vi "Teleop.vi"(10 "Match Info":T3={"Autonomous Elapsed Seconds"=0.0, "TeleOp Elapsed Seconds"=0.0, "Disabled Elapsed Seconds"=0.0, "Visited Autonomous"=FALSE, "Visited TeleOp"=FALSE, "Visited Disabled"=FALSE, "Autonomous Settings"={"Autonomous Style"=enum."Independent", "VI Refnum"=refnum}}, 11 "Call Context":T4) -> ()   [LabVIEW 2016]
doc: "This VI is called for each TeleOp packet received from the DS where the robot is not disabled. It is often used to read from the joysticks and update I/O or to update setpoints for timed control loops. It should complete and return within 20 milliseconds or it may miss DS packets."
uses:
  <vilib>/Rock Robotics/WPI/DriverStation/WPI_DriverStationDerivedRobotMode.ctl
  <vilib>/Rock Robotics/WPI/DriverStation/WPI_DriverStationMatch Info.ctl
  <vilib>/Rock Robotics/Network Tables/NT Read Boolean.vi
  <vilib>/Rock Robotics/Network Tables/NT Read Number.vi
  Robot Global Data.vi
  <vilib>/Rock Robotics/WPI/Utilities/WPI_GetSetVariantRefNum.vi
  <vilib>/Rock Robotics/Network Tables/NT Write Boolean Array.vi
  <vilib>/Rock Robotics/Network Tables/NT Write Numeric Array.vi
  <vilib>/Rock Robotics/Network Tables/NT Write Boolean.vi
  <vilib>/Rock Robotics/WPI/Ultrasonic/WPI_SonarMB1010AnalogRefNum Registry Get.vi
  <vilib>/Rock Robotics/WPI/Ultrasonic/WPI_SonarMB1010AnalogGetRange.vi
  2039lib.lvlib
panel:
  out "Pick Up Roller 2":dbl
  out "Agitator 2":dbl
  out "Speed of Shooter":dbl
  out "Voltage 2":dbl
  out "Voltage":dbl
  out "Toggle 7":bool
  out "Numeric 4":dbl
  out "Numeric 3":dbl
  out "Numeric 2":dbl
  out "Numeric":dbl
  out "PID gains out":T1={"proportional gain (Kc)"=1.0, "integral time (Ti, min)"=0.01, "derivative time (Td, min)"=0.0} {"derivative time (Td, min)" format="%.3f"; "integral time (Ti, min)" format="%.3f"; "proportional gain (Kc)" format="%.3f"}
  in  "PID gains":T1={"proportional gain (Kc)"=1.0, "integral time (Ti, min)"=0.01, "derivative time (Td, min)"=0.0} {"derivative time (Td, min)" format="%.3f"; "integral time (Ti, min)" format="%.3f"; "proportional gain (Kc)" format="%.3f"}
  in  "Teleop State":T2(ring)
  out "Toggle 6":bool
  out "Toggle 5":bool
  out "Toggle 4":bool
  out "Toggle 3":bool
  out "Toggle 2":bool
  out "Sample Slider 0":dbl(slide) scale=0.0..5.0
  out "Sample Boolean 1":bool
  out "Sample Boolean 0":bool
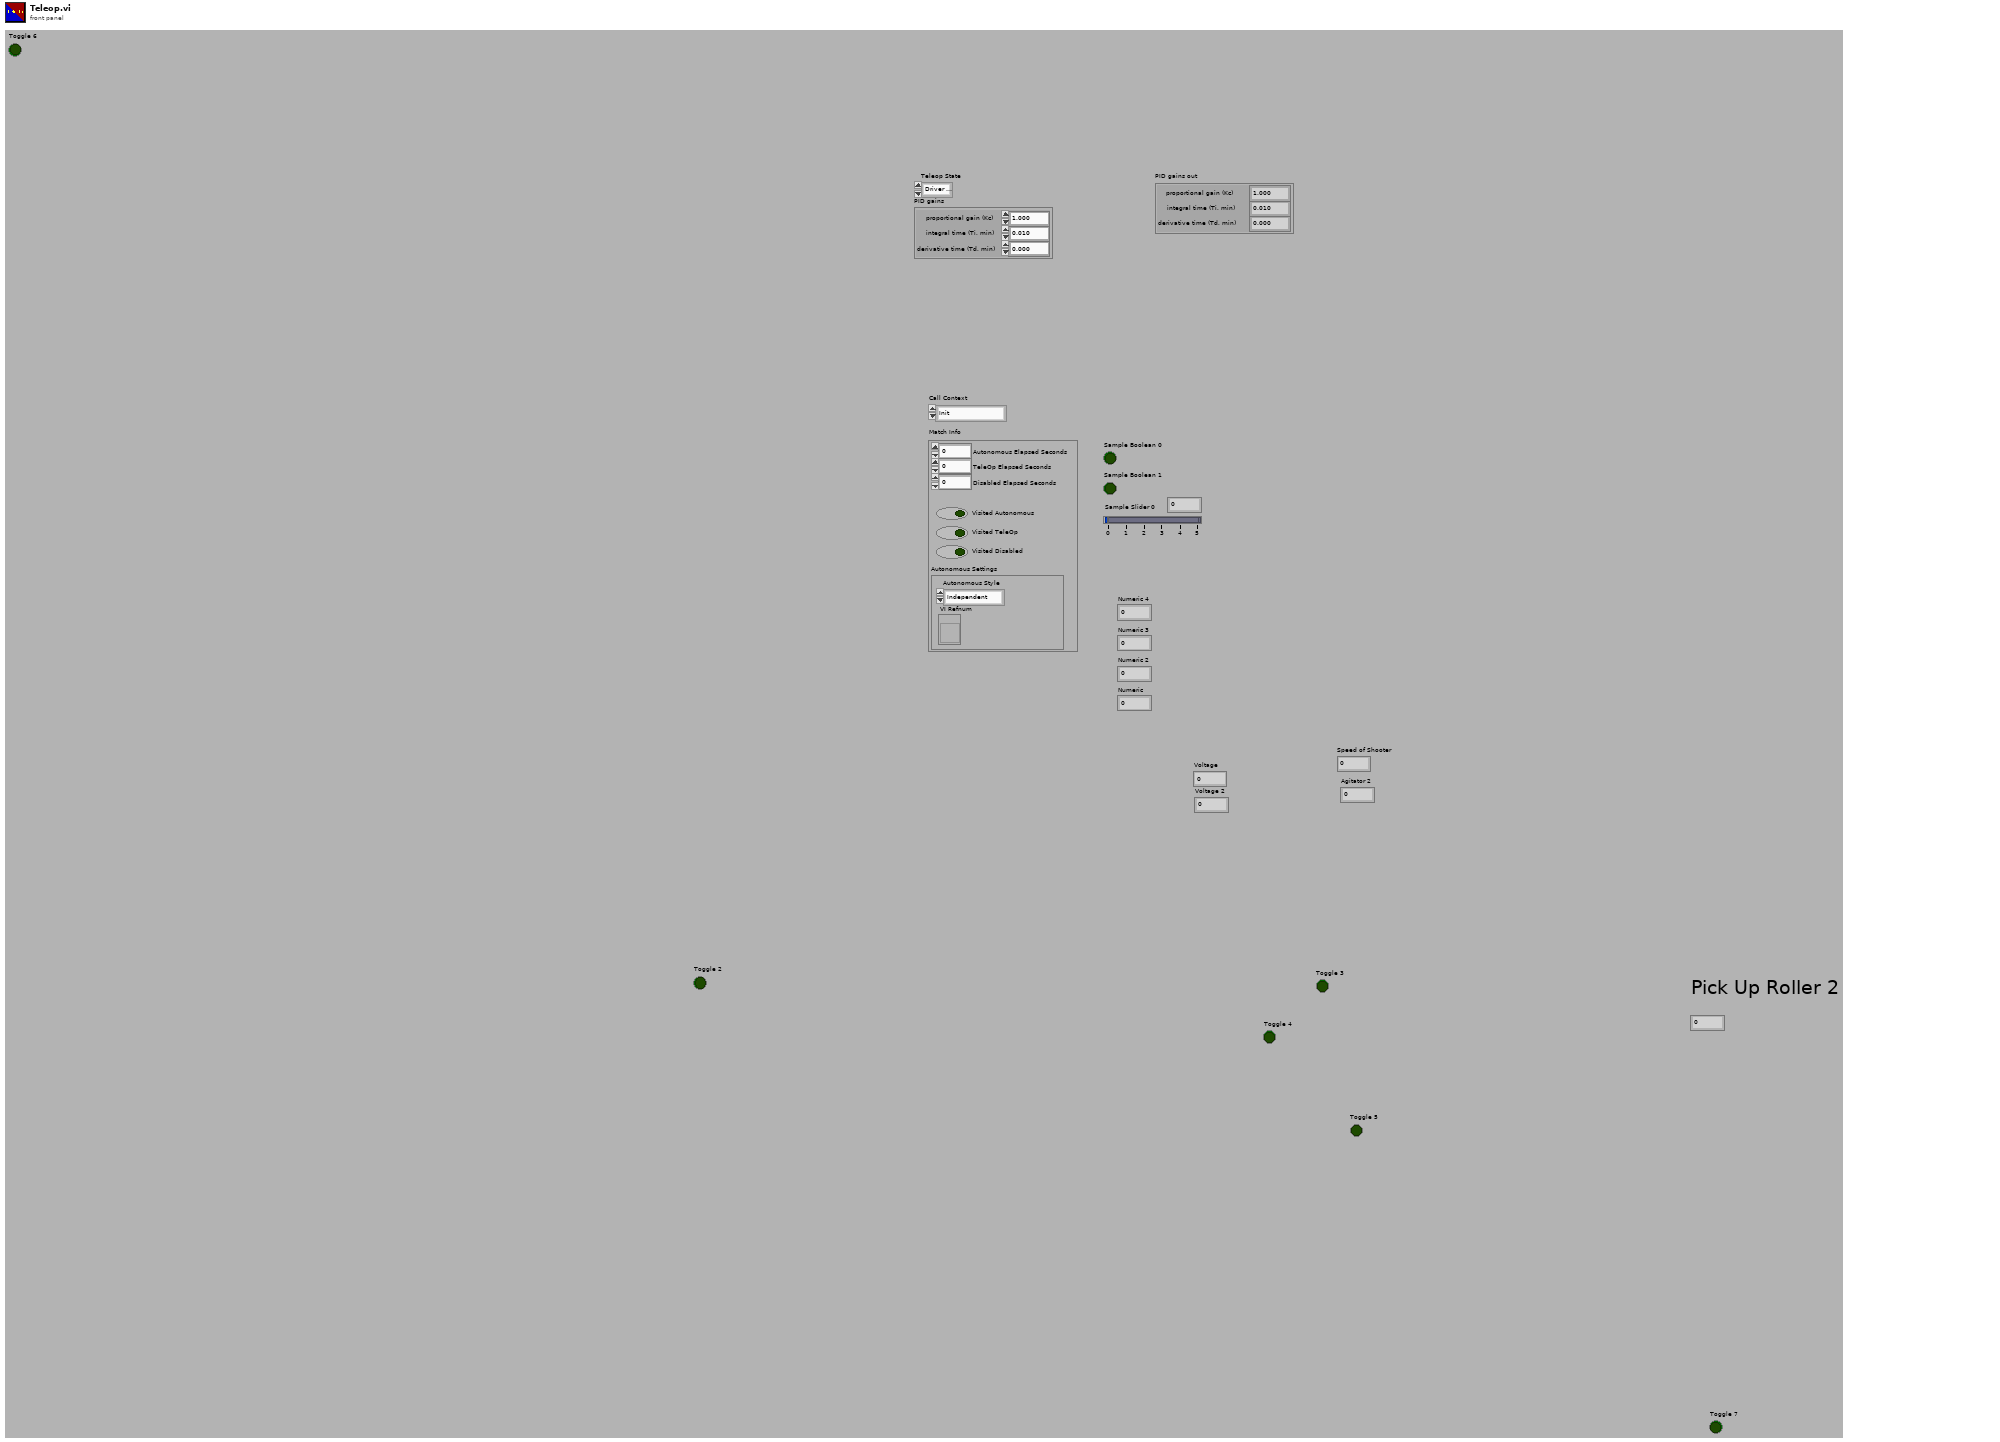
[diagram p1: front panel]
types:
  T1 = cluster{"proportional gain (Kc)":dbl, "integral time (Ti, min)":dbl, "derivative time (Td, min)":dbl}
  T2 = enum16{"Driver Control", "PID Autotune", "Gear Coarse Adjust", "Gear Fine Adjust"}
  T3 = typedef "WPI_DriverStationMatch Info.ctl" = cluster{"Autonomous Elapsed Seconds":dbl, "TeleOp Elapsed Seconds":dbl, "Disabled Elapsed Seconds":dbl, "Visited Autonomous":bool, "Visited TeleOp":bool, "Visited Disabled":bool, "Autonomous Settings":cluster{"Autonomous Style":enum16{"Iterative", "Independent"}, "VI Refnum":refnum<vi>}}
  T4 = typedef "WPI_DriverStationDerivedRobotMode.ctl" = enum16{"Init", "Execute", "Stop"}
  T5 = typedef "WPI_MotorControlDeviceRef.ctl" = cluster{"DeviceStatus":errorcluster, "Type":T6, "PWM":cluster{"PWM Channel":T7, "DeadBand":T8}, "CAN":cluster{"Device Number":u8, "SetOutput VI Ref":variant, "GetOutput VI Ref":variant, "Enable VI Ref":variant, "Disable VI Ref":variant, "Data":variant}, "Invert":bool}
  T6 = typedef "WPI_MotorControlType.ctl" = enum16{"PWM", "CAN"}
  T7 = typedef "FPGA_DIOPWMChannel.ctl" = enum8{"PWM 0", "PWM 1", "PWM 2", "PWM 3", "PWM 4", "PWM 5", "PWM 6", "PWM 7", "PWM 8", "PWM 9", "PWM MXP 0", "PWM MXP 1", "PWM MXP 2", "PWM MXP 3", "PWM MXP 4", "PWM MXP 5", "PWM MXP 6", "PWM MXP 7", "PWM MXP 8", "PWM MXP 9", "Invalid"}
  T8 = typedef "WPI_PWMDeadband.ctl" = cluster{"Name":string, "maxPositivePwm":i32, "minPositivePwm":i32, "centerPwm":i32, "maxNegativePwm":i32, "minNegativePwm":i32, "angularRange":u16}
  T9 = enum16{"Driver Control", "Gear Coarse Adjust", "Gear Fine Adjust"}
  T10 = typedef "WPI_JoystickDevRef.ctl" = cluster{"Device":T11}
  T11 = typedef "WPI_JoystickDeviceEnum.ctl" = enum16{"USB 0", "USB 1", "USB 2", "USB 3", "USB 4", "USB 5"}
  T12 = cluster{"Buttons[0]":bool, "Buttons[1]":bool, "Buttons[2]":bool, "Buttons[3]":bool, "Buttons[4]":bool, "Buttons[5]":bool, "Buttons[6]":bool, "Buttons[7]":bool, "Buttons[8]":bool, "Buttons[9]":bool, "Buttons[10]":bool, "Buttons[11]":bool, "Buttons[12]":bool}
  T13 = typedef "WPI_RobotDriveDevRef.ctl" = cluster{"DevStatus":errorcluster, "Motors[]":T5[], "Square Inputs":bool, "Max Output":dbl}
  T14 = cluster{"Buttons[0]":bool, "Buttons[1]":bool, "Buttons[2]":bool, "Buttons[3]":bool, "Buttons[4]":bool, "Buttons[5]":bool, "Buttons[6]":bool, "Buttons[7]":bool, "Buttons[8]":bool}
  T15 = typedef "WPI_ServoDeviceRef.ctl" = cluster{"DeviceStatus":errorcluster, "PWM Channel":T7, "DeadBand":T8}
  T16 = typedef "WPI_SonarMB1010AnalogDeviceRef.ctl" = cluster{"AIDeviceRef":T17, "Scaling factor (V/in)":dbl, "Average Bits":u8}
  T17 = typedef "WPI_AnalogChannelDevRef.ctl" = cluster{"DevStatus":errorcluster, "Analog Channel":T18}
  T18 = typedef "FPGA_AIChannel.ctl" = enum8{"AI 0", "AI 1", "AI 2", "AI 3", "AI MXP 0", "AI MXP 1", "AI MXP 2", "AI MXP 3", "Invalid"}
  T19 = typedef "WPI_DigitalInputDevRef.ctl" = cluster{"DevStatus":errorcluster, "DIO Channel":T20}
  T20 = typedef "FPGA_DIOChannel.ctl" = enum8{"DIO 0", "DIO 1", "DIO 2", "DIO 3", "DIO 4", "DIO 5", "DIO 6", "DIO 7", "DIO 8", "DIO 9", "DIO MXP 0", "DIO MXP 1", "DIO MXP 2", "DIO MXP 3", "DIO MXP 4", "DIO MXP 5", "DIO MXP 6", "DIO MXP 7", "DIO MXP 8", "DIO MXP 9", "DIO MXP 10", "DIO MXP 11", "DIO MXP 12", "DIO MXP 13", "DIO MXP 14", "DIO MXP 15", "SPI Port CS1", "SPI Port CS2", "SPI Port CS3", "SPI Port MISO", "SPI Port MOSI", "Invalid"}
  T21 = typedef "WPI_SwitchDevRef.ctl" = cluster{"DevStatus":errorcluster, "DIO Channel":T20, "CntIndex":T22, "Normally Closed":bool}
  T22 = typedef "FPGA_CounterCtrSystemIndex.ctl" = enum8{"Ctr 0", "Ctr 1", "Ctr 2", "Ctr 3", "Ctr 4", "Ctr 5", "Ctr 6", "Ctr 7", "Invalid"}
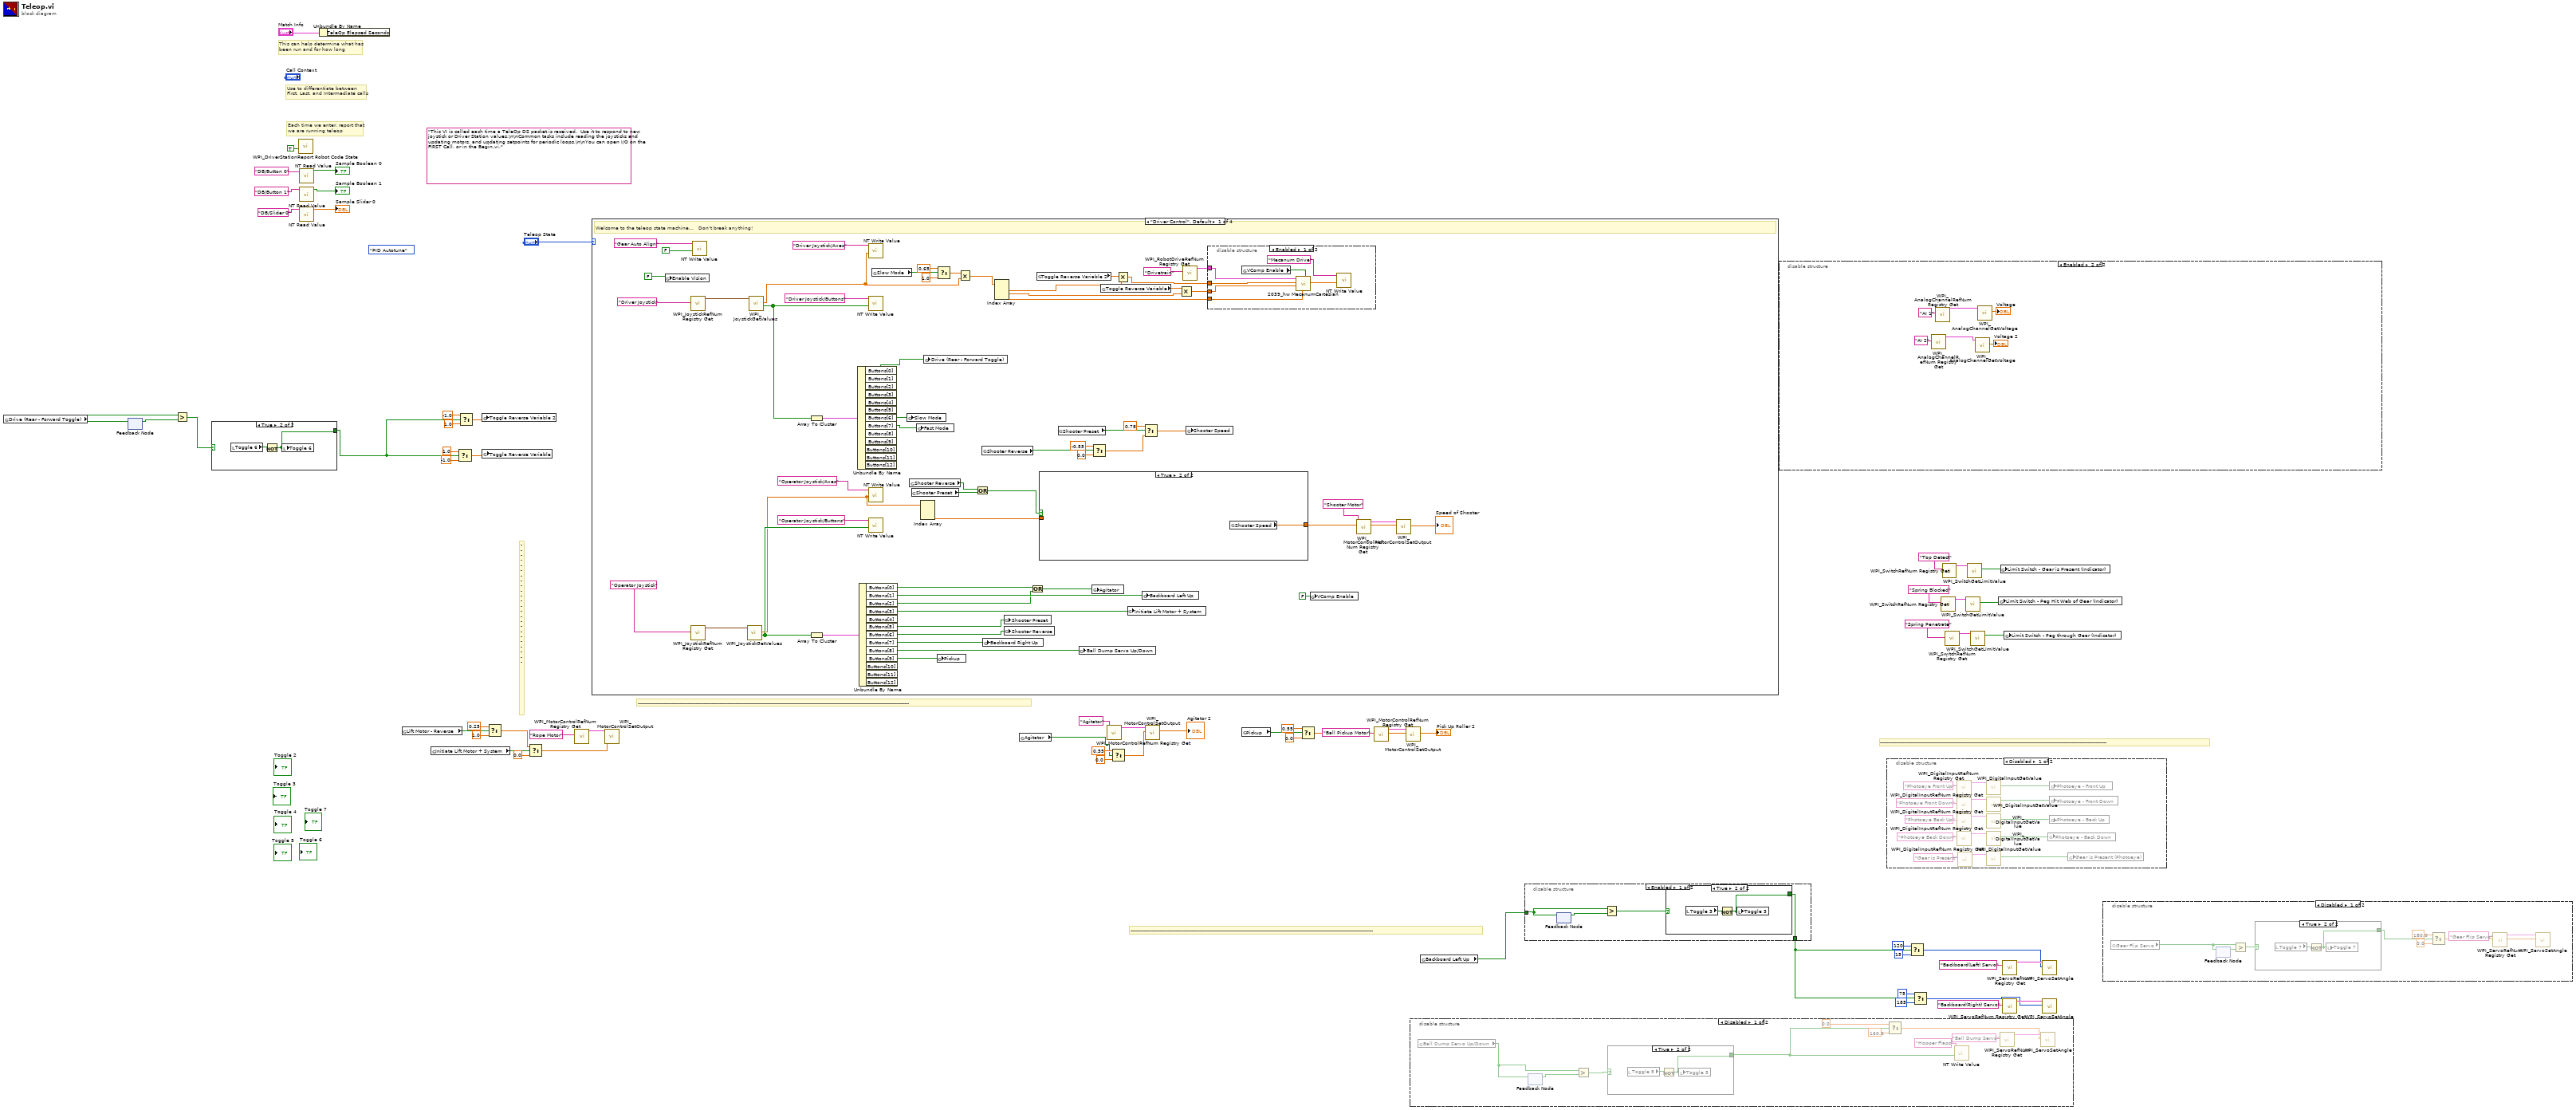
[diagram p0: block diagram]
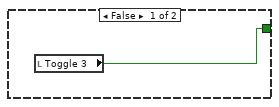
[diagram p3: hidden frame]
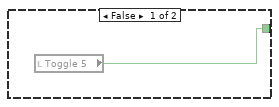
[diagram p5: hidden frame]
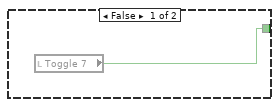
[diagram p7: hidden frame]
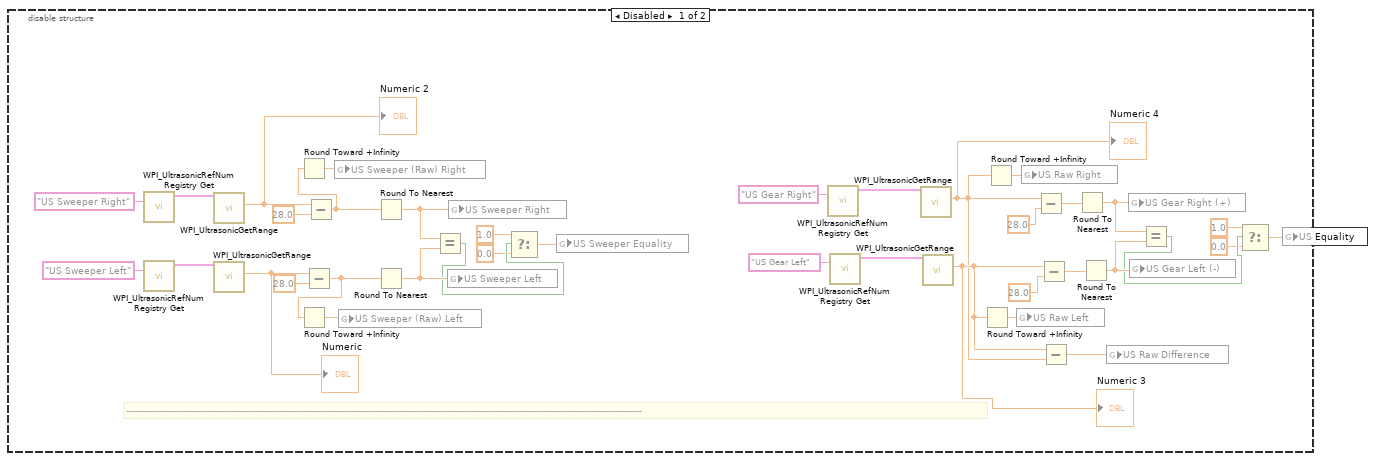
[diagram p9: hidden frame]
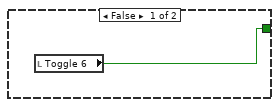
[diagram p10: hidden frame]
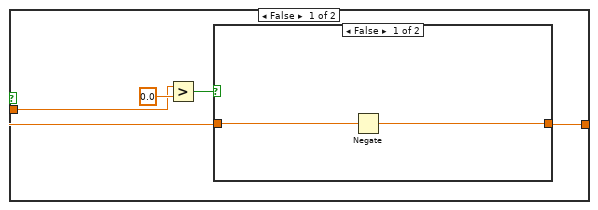
[diagram p11: hidden frame]
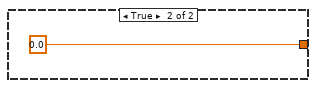
[diagram p12: hidden frame]
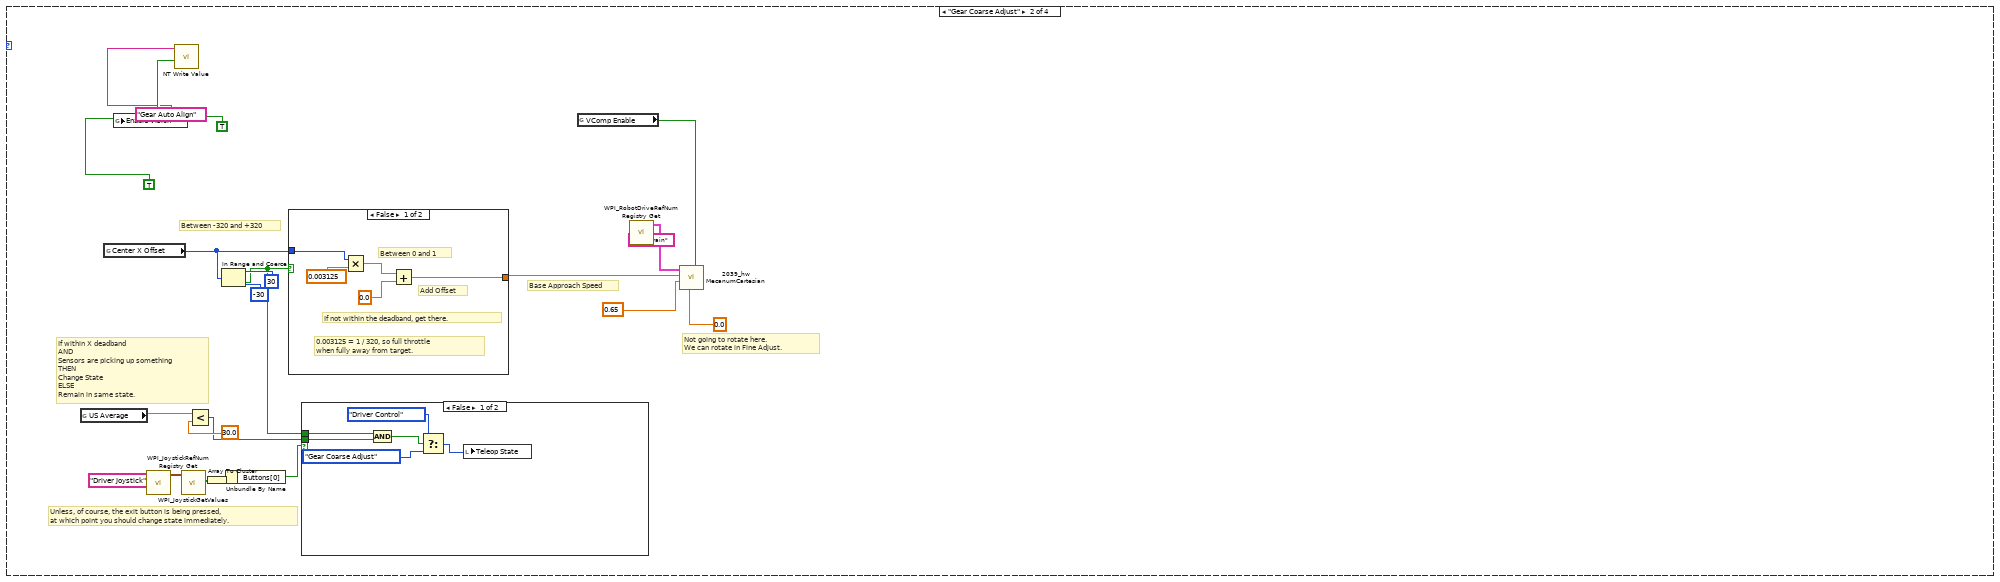
[diagram p14: hidden frame]
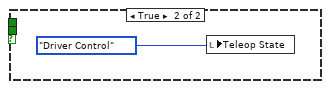
[diagram p15: hidden frame]
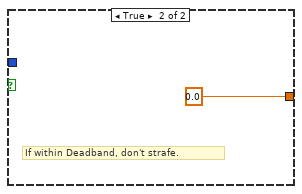
[diagram p16: hidden frame]
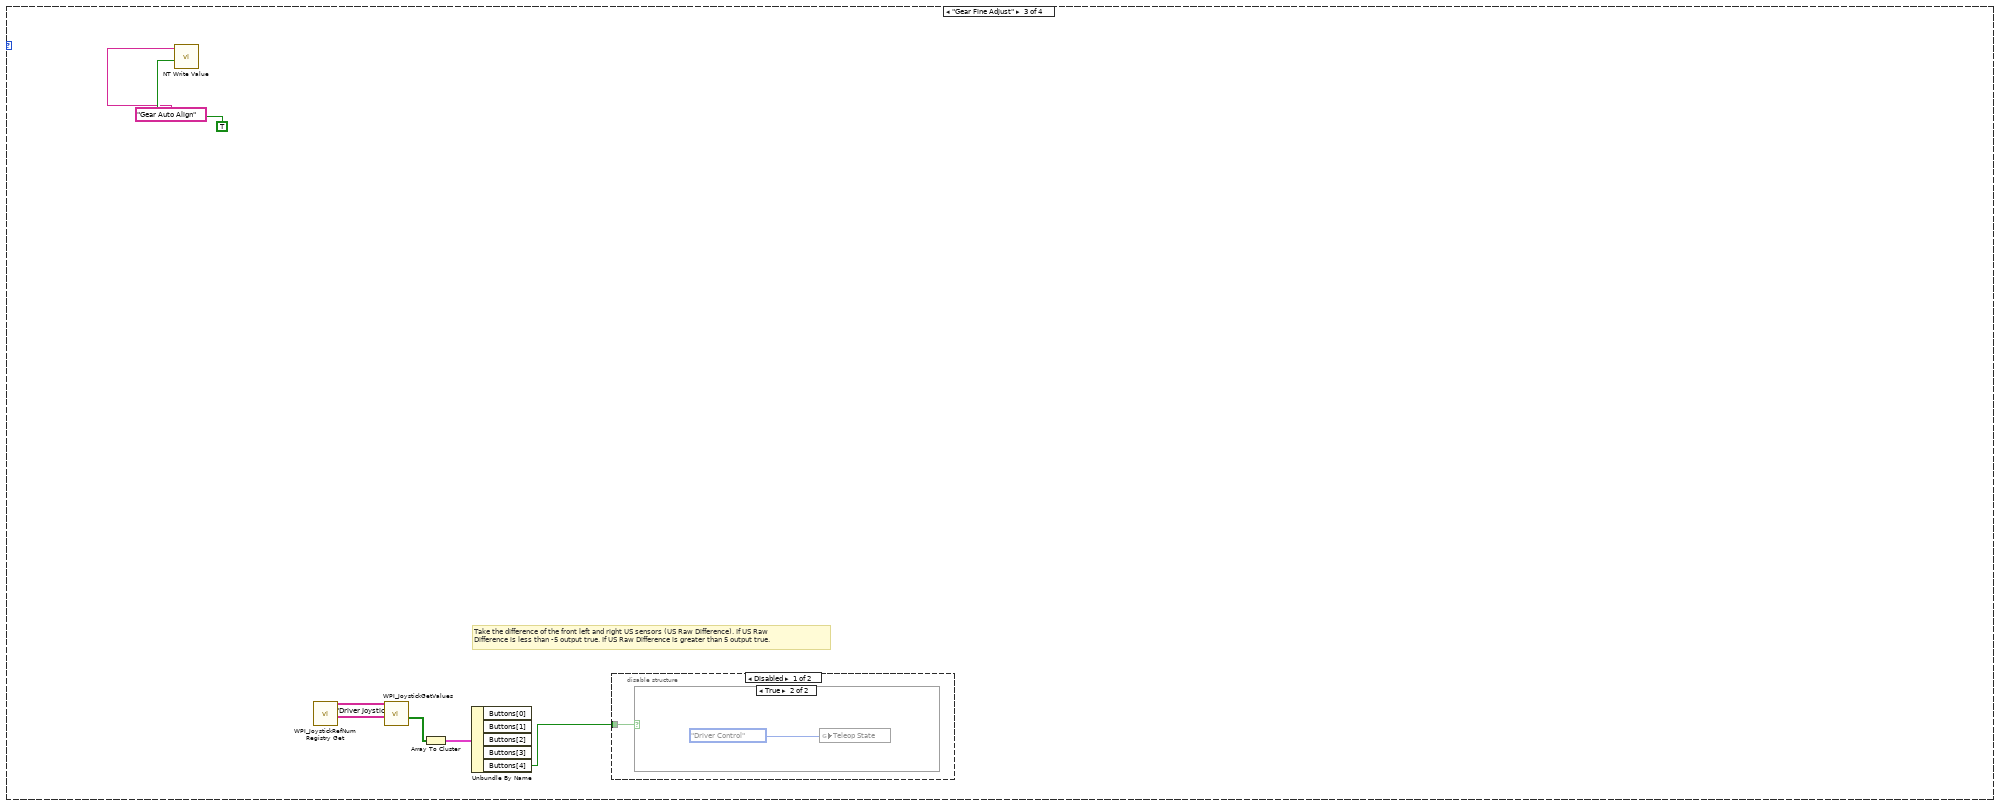
[diagram p17: hidden frame]
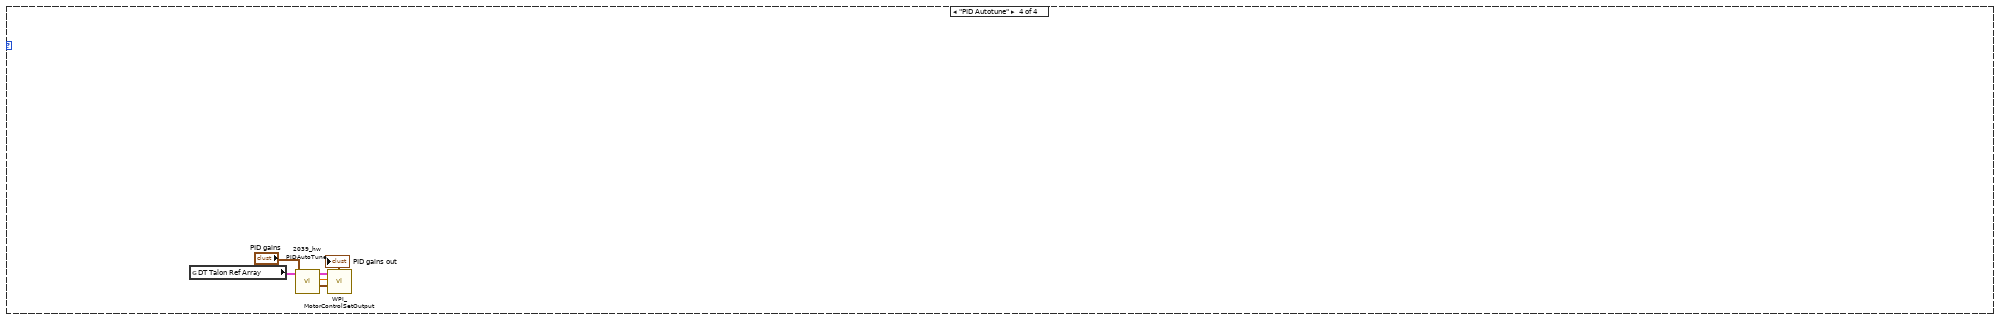
[diagram p20: hidden frame]
diagram:
  (unwired) T2."PID Autotune" ("Teleop State")
  (unwired) "This VI is called each time a TeleOp DS packet is received.  Use it to respond to new joystick or Driver Station values.\n\nCommon tasks include reading the joysticks and updating motors, and updating setpoints for periodic loops.\n\nYou can open I/O on the FIRST Call, or in the Begin.vi."
  # "-\n-\n-\n-\n-\n-\n-\n-\n-\n-\n-\n-\n-\n-\n-\n-\n-\n-\n-\n-\n-\n-\n-\n-"
  # "--------------------------------------------------------------------------------------------------------------------------------------------------------------------------"
  # "--------------------------------------------------------------------------------------------------------------------------------------------------------"
  # "----------------------------------------------------------------------------------------------------------------------------------------------"
  # "Each time we enter, report that\nwe are running teleop"
  # "Use to differentiate between\nFirst, Last, and Intermediate calls"
  # "This can help determine what has\nbeen run and for how long"
  n1 = global read "Robot Global Data.vi" "Drive (Rear - Forward Toggle)"() -> (w3:bool)
  n2 = feedback #1() -> (w35:bool)  [unwired: 1 in]
  n3 = feedback-in #1(w3) -> ()
  n4 = Greater?(x=w3, y=w35) -> (0:w34:bool)
  n5 = case shown="True" w34 {
    tunnel: [w64 w65] -> w7
    frame False {
      n6 = local read "Toggle 6"() -> (w64:bool)
    }
    frame True {
      n7 = local read "Toggle 6"() -> (w66:bool)
      n8 = Not(x=w66) -> (.not. x?=w65:bool)
      n9 = local write "Toggle 6"(w65) -> ()
    }
  }
  n10 = call <vilib>:"WPI_DriverStationReport Robot Code State.vi"("TeleOp"=TRUE ("Autonomous")) -> ()  [unwired: 10 in, 1 out]
  n11 = call-poly <vilib>:"NT Read Value.vi"("Name"="DB/Button 0" ("refnum name")) -> ("Boolean"=→"Sample Boolean 0":bool)  [unwired: 9 in, 1 out]
  n12 = call-poly <vilib>:"NT Read Value.vi"("Name"="DB/Button 1" ("refnum name")) -> ("Boolean"=→"Sample Boolean 1":bool)  [unwired: 9 in, 1 out]
  n13 = call-poly <vilib>:"NT Read Value.vi"("Name"="DB/Slider 0" ("refnum name")) -> ("Numeric"=→"Sample Slider 0":dbl)  [unwired: 9 in, 1 out]
  n14 = Unbundle By Name("Match Info") -> ()  [unwired: 1 out]
  n15 = global read "Robot Global Data.vi" "Lift Motor - Reverse"() -> (w26:bool)
  n16 = global read "Robot Global Data.vi" "Initiate Lift Motor + System"() -> (w31:bool)
  n17 = Select(t=1.0, s=w7, f=-1.0) -> (s? t:f=w44:dbl)
  n18 = Select(t=-1.0, s=w7, f=1.0) -> (s? t:f=w10:dbl)
  n19 = global write "Robot Global Data.vi" "Toggle Reverse Variable 2"(w10) -> ()
  n20 = global write "Robot Global Data.vi" "Toggle Reverse Variable"(w44) -> ()
  n21 = Select(t=0.25, s=w26, f=1.0) -> (s? t:f=w29:dbl)
  n22 = Select(t=w29, s=w31, f=0.0) -> (s? t:f=w36:dbl)
  n23 = call <vilib>:"WPI_MotorControlRefNum Registry Get.vi"("refnum name"="Rope Motor") -> ("MotorControlDevRef"=w48:T5)  [unwired: 9 in, 1 out]
  n24 = case shown="\"Driver Control\", Default" "Teleop State" {
    frame "Driver Control", Default {
      # "Welcome to the teleop state machine...   Don't break anything!"
      n25 = global write "Robot Global Data.vi" "Enable Vision"(FALSE) -> ()
      n26 = call <vilib>:"WPI_JoystickRefNum Registry Get.vi"("refnum name"="Driver Joystick") -> ("JoystickDevRef"=w123:T10)  [unwired: 1 in, 9 out]
      n27 = call <vilib>:"WPI_JoystickRefNum Registry Get.vi"("refnum name"="Operator Joystick") -> ("JoystickDevRef"=w118:T10)  [unwired: 9 in, 1 out]
      n28 = call-poly <vilib>:"NT Write Value.vi"("Boolean"=FALSE, "Name"="Gear Auto Align") -> ()  [unwired: 9 in, 1 out]
      n29 = call <vilib>:"WPI_JoystickGetValues.vi"("JoystickDevRef"=w118) -> ("Buttons"=w115:bool[], "Axes"=w94:dbl[])  [unwired: 6 in, 3 out]
      n30 = call <vilib>:"WPI_JoystickGetValues.vi"("JoystickDevRef"=w123) -> ("Buttons"=w120:bool[], "Axes"=w97:dbl[])  [unwired: 6 in, 3 out]
      n31 = Array To Cluster(array=w120) -> (cluster=w111:T12)
      n32 = Array To Cluster(array=w115) -> (cluster=w112:T12)
      n33 = Unbundle By Name(w111) -> ("Buttons[0]"=w110:bool, "Buttons[6]"=w107:bool, "Buttons[7]"=w104:bool)  [unwired: 10 out]
      n34 = Unbundle By Name(w112) -> ("Buttons[0]"=w71:bool, "Buttons[1]"=w90:bool, "Buttons[2]"=w72:bool, "Buttons[3]"=w87:bool, "Buttons[5]"=w85:bool, "Buttons[6]"=w84:bool, "Buttons[7]"=w109:bool, "Buttons[8]"=w108:bool, "Buttons[9]"=w67:bool)  [unwired: 4 out]
      n35 = call-poly <vilib>:"NT Write Value.vi"("Numeric Array"=w97, "Name"="Driver Joystick/Axes") -> ()  [unwired: 9 in, 1 out]
      n36 = call-poly <vilib>:"NT Write Value.vi"("Boolean Array"=w120, "Name"="Driver Joystick/Buttons") -> ()  [unwired: 9 in, 1 out]
      n37 = call-poly <vilib>:"NT Write Value.vi"("Numeric Array"=w94, "Name"="Operator Joystick/Axes") -> ()  [unwired: 9 in, 1 out]
      n38 = call-poly <vilib>:"NT Write Value.vi"("Boolean Array"=w115, "Name"="Operator Joystick/Buttons") -> ()  [unwired: 9 in, 1 out]
      n39 = global read "Robot Global Data.vi" "Slow Mode"() -> (w101:bool)
      n40 = global write "Robot Global Data.vi" "Slow Mode"(w107) -> ()
      n41 = global read "Robot Global Data.vi" "Shooter Reverse"() -> (w75:bool)
      n42 = global read "Robot Global Data.vi" "Shooter Preset"() -> (w76:bool)
      n43 = global write "Robot Global Data.vi" "Fast Mode"(w104) -> ()
      n44 = Index Array(array=w94) -> (element #3=w88:dbl)  [unwired: 3 in, 2 out]
      n45 = global write "Robot Global Data.vi" "Drive (Rear - Forward Toggle)"(w110) -> ()
      n46 = Select(t=0.65, s=w101, f=1.0) -> (s? t:f=w98:dbl)
      n47 = global write "Robot Global Data.vi" "Pickup"(w67) -> ()
      n48 = Multiply(x=w98, y=w97) -> (x*y=w96:dbl[])
      n49 = Or(x=w75, y=w76) -> (x .or. y?=w74:bool)
      n50 = global read "Robot Global Data.vi" "Shooter Reverse"() -> (w80:bool)
      n51 = global write "Robot Global Data.vi" "Backboard Right Up"(w109) -> ()
      n52 = Index Array(array=w96) -> (element #1=w69:dbl, element #2=w103:dbl, element #3=w102:dbl)  [unwired: 3 in]
      n53 = global write "Robot Global Data.vi" "Shooter Preset"(w85) -> ()
      n54 = global write "Robot Global Data.vi" "Shooter Reverse"(w84) -> ()
      n55 = Or(x=w71, y=w72) -> (x .or. y?=w73:bool)
      n56 = global read "Robot Global Data.vi" "Toggle Reverse Variable 2"() -> (w70:dbl)
      n57 = case shown="True" w74 {
        tunnel: [w128 w134] -> w89
        tunnel: w88 -> [w127 _]
        frame False {
          n58 = Greater?(x=w127, y=0.0) -> (0:w129:bool)
          n59 = case shown="False" w129 {
            tunnel: [w131 0.0 ("y")] -> w128
            tunnel: w127 -> [w132 _]
            frame False {
              n60 = Negate(x=w132) -> (-x=w131:dbl)
            }
            frame True {
            }
          }
        }
        frame True {
          n61 = global read "Robot Global Data.vi" "Shooter Speed"() -> (w134:dbl)
        }
      }
      n62 = global read "Robot Global Data.vi" "Shooter Preset"() -> (w83:bool)
      n63 = global write "Robot Global Data.vi" "Ball Dump Servo Up/Down"(w108) -> ()
      n64 = Select(t=-0.55, s=w80, f=0.0) -> (s? t:f=w77:dbl)
      n65 = global write "Robot Global Data.vi" "Agitator"(w73) -> ()
      n66 = global read "Robot Global Data.vi" "Toggle Reverse Variable"() -> (w113:dbl)
      n67 = Multiply(x=w70, y=w69) -> (x*y=w68:dbl)
      n68 = global write "Robot Global Data.vi" "Initiate Lift Motor + System"(w87) -> ()
      n69 = global write "Robot Global Data.vi" "Backboard Left Up"(w90) -> ()
      n70 = Select(t=0.78, s=w83, f=w77) -> (s? t:f=w81:dbl)
      n71 = Multiply(x=w113, y=w103) -> (x*y=w114:dbl)
      n72 = call <vilib>:"WPI_RobotDriveRefNum Registry Get.vi"("refnum name"="Drivetrain") -> ("RobotDriveDevRef"=w125:T13)  [unwired: 1 in, 9 out]
      n73 = global write "Robot Global Data.vi" "Shooter Speed"(w81) -> ()
      n74 = disable-structure shown="Enabled" {
        disable-tunnel: w125 -> [w141 _]
        disable-tunnel: w114 -> [w138 _]
        disable-tunnel: w102 -> [w135 _]
        disable-tunnel: w68 -> [w136 _]
        frame Enabled {
          n75 = global read "Robot Global Data.vi" "VComp Enable"() -> (w137:bool)
          n76 = call "2039_hw MecanumCartesian.vi"("VComp Scaling"=w137, "Rotation"=w135, "Y"=w138, "X"=w136, "RobotDriveDevRef"=w141) -> ("Motor Values"=w139:dbl[])  [unwired: 4 in, 2 out]
          n77 = call-poly <vilib>:"NT Write Value.vi"("Numeric Array"=w139, "Name"="Mecanum Drive") -> ()  [unwired: 9 in, 1 out]
        }
        frame Disabled {
        }
      }
      n78 = global write "Robot Global Data.vi" "VComp Enable"(FALSE ("VComp Enable")) -> ()
      n79 = call <vilib>:"WPI_MotorControlRefNum Registry Get.vi"("refnum name"="Shooter Motor") -> ("MotorControlDevRef"=w92:T5)  [unwired: 9 in, 1 out]
      n80 = call <vilib>:"WPI_MotorControlSetOutput.vi"("Output"=w89, "MotorControlDevRef"=w92) -> ("Motor Output"=→"Speed of Shooter":dbl)  [unwired: 7 in, 2 out]
    }
    frame "Gear Coarse Adjust" {
      # "Base Approach Speed"
      # "If within X deadband\nAND\nSensors are picking up something\nTHEN\nChange State\nELSE\nRemain in same state."
      # "Unless, of course, the exit button is being pressed, \nat which point you should change state immediately."
      # "Not going to rotate here.\nWe can rotate in Fine Adjust."
      # "Between -320 and +320"
      n81 = global read "Robot Global Data.vi" "US Average"() -> (w150:dbl)
      n82 = global read "Robot Global Data.vi" "Center X Offset"() -> (w159:i32)
      n83 = global write "Robot Global Data.vi" "Enable Vision"(TRUE) -> ()
      n84 = call <vilib>:"WPI_JoystickRefNum Registry Get.vi"("refnum name"="Driver Joystick") -> ("JoystickDevRef"=w146:T10)  [unwired: 1 in, 9 out]
      n85 = call-poly <vilib>:"NT Write Value.vi"("Boolean"=TRUE, "Name"="Gear Auto Align") -> ()  [unwired: 9 in, 1 out]
      n86 = call <vilib>:"WPI_JoystickGetValues.vi"("JoystickDevRef"=w146) -> ("Buttons"=w145:bool[])  [unwired: 6 in, 4 out]
      n87 = Less?(x=w150, y=30.0) -> (x < y?=w148:bool)
      n88 = Array To Cluster(array=w145) -> (cluster=w144:T14)
      n89 = In Range and Coerce(upper limit=30, x=w159, lower limit=-30) -> (In Range?=w151:bool)  [unwired: 1 out]
      n90 = Unbundle By Name(w144) -> ("Buttons[0]"=w143:bool)
      n91 = case shown="False" w151 {
        tunnel: w159 -> [w174 _]
        tunnel: [w170 0.0] -> w156
        frame False {
          # "0.003125 = 1 / 320, so full throttle\nwhen fully away from target."
          # "If not within the deadband, get there."
          # "Add Offset"
          # "Between 0 and 1"
          n92 = Multiply(x=w174, y=0.003125) -> (x*y=w172:dbl)
          n93 = Add(x=w172, y=0.0) -> (x+y=w170:dbl)
        }
        frame True {
          # "If within Deadband, don't strafe."
        }
      }
      n94 = case shown="False" w143 {
        tunnel: w151 -> [w168 _]
        tunnel: w148 -> [w167 _]
        frame False {
          n95 = And(x=w168, y=w167) -> (x .and. y?=w164:bool)
          n96 = Select(t=T2."Driver Control" ("Teleop State"), s=w164, f=T2."Gear Coarse Adjust" ("Teleop State")) -> (s? t:f=w163:T2)
          n97 = local write "Teleop State"(w163) -> ()
        }
        frame True {
          n98 = local write "Teleop State"(T2."Driver Control" ("Teleop State")) -> ()
        }
      }
      n99 = global read "Robot Global Data.vi" "VComp Enable"() -> (w152:bool)
      n100 = call <vilib>:"WPI_RobotDriveRefNum Registry Get.vi"("refnum name"="Drivetrain") -> ("RobotDriveDevRef"=w154:T13)  [unwired: 1 in, 9 out]
      n101 = call "2039_hw MecanumCartesian.vi"("VComp Scaling"=w152, "Rotation"=0.0, "Y"=0.65, "X"=w156, "RobotDriveDevRef"=w154) -> ()  [unwired: 4 in, 3 out]
    }
    frame "Gear Fine Adjust" {
      # "Take the difference of the front left and right US sensors (US Raw Difference). If US Raw \nDifference is less than -5 output true. If US Raw Difference is greater than 5 output true."
      n102 = call-poly <vilib>:"NT Write Value.vi"("Boolean"=TRUE, "Name"="Gear Auto Align") -> ()  [unwired: 9 in, 1 out]
      n103 = call <vilib>:"WPI_JoystickRefNum Registry Get.vi"("refnum name"="Driver Joystick") -> ("JoystickDevRef"=w180:T10)  [unwired: 9 in, 1 out]
      n104 = call <vilib>:"WPI_JoystickGetValues.vi"("JoystickDevRef"=w180) -> ("Buttons"=w179:bool[])  [unwired: 6 in, 4 out]
      n105 = Array To Cluster(array=w179) -> (cluster=w178:T14)
      n106 = Unbundle By Name(w178) -> ("Buttons[4]"=w177:bool)  [unwired: 4 out]
      n107 = disable-structure shown="Disabled" {
        disable-tunnel: w177 -> [w183 _]
        frame Disabled {
          n108 = case shown="True" w183 {
            frame False {
            }
            frame True {
              n109 = global write "Robot Global Data.vi" "Teleop State"(T9."Driver Control") -> ()
            }
          }
        }
        frame Enabled {
        }
      }
    }
    frame "PID Autotune" {
      n110 = global read "Robot Global Data.vi" "DT Talon Ref Array"() -> (w189:T5[])
      n111 = call "2039_hw PIDAutoTune.vi"("PID gains"="PID gains", "CAN Talon SRX Ref"=w189) -> ("PID gains out"=→"PID gains out":T1, "To Motors"=w187:dbl, "Tuning Talon"=w188:T5)  [unwired: 7 in]
      n112 = call <vilib>:"WPI_MotorControlSetOutput.vi"("Output"=w187, "MotorControlDevRef"=w188) -> ()  [unwired: 7 in, 3 out]
    }
  }
  n113 = call <vilib>:"WPI_MotorControlSetOutput.vi"("Output"=w36, "MotorControlDevRef"=w48) -> ()  [unwired: 7 in, 3 out]
  n114 = global read "Robot Global Data.vi" "Agitator"() -> (w18:bool)
  n115 = call <vilib>:"WPI_MotorControlRefNum Registry Get.vi"("refnum name"="Agitator") -> ("MotorControlDevRef"=w24:T5)  [unwired: 9 in, 1 out]
  n116 = Select(t=0.55, s=w18, f=0.0) -> (s? t:f=w22:dbl)
  n117 = call <vilib>:"WPI_MotorControlSetOutput.vi"("Output"=w22, "MotorControlDevRef"=w24) -> ("Motor Output"=→"Agitator 2":dbl)  [unwired: 7 in, 2 out]
  n118 = global read "Robot Global Data.vi" "Pickup"() -> (w11:bool)
  n119 = Select(t=0.55, s=w11, f=0.0) -> (s? t:f=w14:dbl)
  n120 = call <vilib>:"WPI_MotorControlRefNum Registry Get.vi"("refnum name"="Ball Pickup Motor") -> ("MotorControlDevRef"=w17:T5)  [unwired: 9 in, 1 out]
  n121 = call <vilib>:"WPI_MotorControlSetOutput.vi"("Output"=w14, "MotorControlDevRef"=w17) -> ("Motor Output"=→"Pick Up Roller 2":dbl)  [unwired: 7 in, 2 out]
  n122 = disable-structure shown="Disabled" {
    frame Disabled {
      n123 = global read "Robot Global Data.vi" "Ball Dump Servo Up/Down"() -> (w194:bool)
      n124 = feedback #2() -> (w196:bool)  [unwired: 1 in]
      n125 = feedback-in #2(w194) -> ()
      n126 = Greater?(x=w194, y=w196) -> (0:w195:bool)
      n127 = case shown="True" w195 {
        tunnel: [w200 w201] -> w191
        frame False {
          n128 = local read "Toggle 5"() -> (w200:bool)
        }
        frame True {
          n129 = local read "Toggle 5"() -> (w202:bool)
          n130 = Not(x=w202) -> (.not. x?=w201:bool)
          n131 = local write "Toggle 5"(w201) -> ()
        }
      }
      n132 = Select(t=0.0 ("Ball Dump Servo (Up)"), s=w191, f=160.0) -> (s? t:f=w190:dbl)
      n133 = call-poly <vilib>:"NT Write Value.vi"("Boolean"=w191, "Name"="Hopper Flaps") -> ()  [unwired: 9 in, 1 out]
      n134 = call <vilib>:"WPI_ServoRefNum Registry Get.vi"("refnum name"="Ball Dump Servo") -> ("ServoDeviceRef"=w199:T15)  [unwired: 9 in, 1 out]
      n135 = call <vilib>:"WPI_ServoSetAngle.vi"("Angle"=w190, "ServoDeviceRef"=w199) -> ()  [unwired: 8 in, 2 out]
    }
    frame Enabled {
    }
  }
  n136 = global read "Robot Global Data.vi" "Backboard Left Up"() -> (w2:bool)
  n137 = disable-structure shown="Enabled" {
    disable-tunnel: w2 -> [w204 _]
    disable-tunnel: [w203 _] -> w1
    frame Enabled {
      n138 = feedback #3() -> (w206:bool)  [unwired: 1 in]
      n139 = feedback-in #3(w204) -> ()
      n140 = Greater?(x=w204, y=w206) -> (0:w205:bool)
      n141 = case shown="True" w205 {
        tunnel: [w207 w208] -> w203
        frame False {
          n142 = local read "Toggle 3"() -> (w207:bool)
        }
        frame True {
          n143 = local read "Toggle 3"() -> (w209:bool)
          n144 = Not(x=w209) -> (.not. x?=w208:bool)
          n145 = local write "Toggle 3"(w208) -> ()
        }
      }
    }
    frame Disabled {
    }
  }
  n146 = disable-structure shown="Enabled" {
    frame Disabled {
      # "----------------------------------------------------------------------------------------------------------------------------------------------------------------------------"
      n147 = call-poly <vilib>:"WPI_UltrasonicRefNum Registry Get.vi"("refnum name"="US Sweeper Right") -> ("SonarMB1010AnalogDevRef"=w227:T16)  [unwired: 9 in, 1 out]
      n148 = call-poly <vilib>:"WPI_UltrasonicRefNum Registry Get.vi"("refnum name"="US Sweeper Left") -> ("SonarMB1010AnalogDevRef"=w228:T16)  [unwired: 9 in, 1 out]
      n149 = call-poly <vilib>:"WPI_UltrasonicGetRange.vi"("SonarMB1010AnalogDevRef"=w227) -> ("Distance"=w212:dbl)  [unwired: 8 in, 2 out]
      "Numeric 2" <- w212
      n150 = call-poly <vilib>:"WPI_UltrasonicGetRange.vi"("SonarMB1010AnalogDevRef"=w228) -> ("Distance"=w213:dbl)  [unwired: 8 in, 2 out]
      "Numeric" <- w213
      n151 = Subtract(x=w213, y=28.0) -> (x-y=w214:dbl)
      n152 = Round Toward +Infinity(x=w214) -> (ceil(x): smallest int >= x=w224:dbl)
      n153 = Subtract(x=w212, y=28.0) -> (x-y=w215:dbl)
      n154 = Round Toward +Infinity(x=w215) -> (ceil(x): smallest int >= x=w223:dbl)
      n155 = global write "Robot Global Data.vi" "US Sweeper (Raw) Right"(w223) -> ()
      n156 = global write "Robot Global Data.vi" "US Sweeper (Raw) Left"(w224) -> ()
      n157 = Round To Nearest(number=w215) -> (nearest integer value=w221:dbl)
      n158 = Round To Nearest(number=w214) -> (nearest integer value=w222:dbl)
      n159 = Equal?(x=w221, y=w222) -> (x = y?=w220:bool)
      n160 = global write "Robot Global Data.vi" "US Sweeper Left"(w222) -> ()
      n161 = global write "Robot Global Data.vi" "US Sweeper Right"(w221) -> ()
      n162 = Select(t=1.0, s=w220, f=0.0) -> (s? t:f=w217:dbl)
      n163 = global write "Robot Global Data.vi" "US Sweeper Equality"(w217) -> ()
      n164 = call-poly <vilib>:"WPI_UltrasonicRefNum Registry Get.vi"("refnum name"="US Gear Right") -> ("SonarMB1010AnalogDevRef"=w245:T16)  [unwired: 9 in, 1 out]
      n165 = call-poly <vilib>:"WPI_UltrasonicRefNum Registry Get.vi"("refnum name"="US Gear Left") -> ("SonarMB1010AnalogDevRef"=w243:T16)  [unwired: 9 in, 1 out]
      n166 = call-poly <vilib>:"WPI_UltrasonicGetRange.vi"("SonarMB1010AnalogDevRef"=w245) -> ("Distance"=w210:dbl)  [unwired: 8 in, 2 out]
      "Numeric 4" <- w210
      n167 = call-poly <vilib>:"WPI_UltrasonicGetRange.vi"("SonarMB1010AnalogDevRef"=w243) -> ("Distance"=w211:dbl)  [unwired: 8 in, 2 out]
      "Numeric 3" <- w211
      n168 = Round Toward +Infinity(x=w211) -> (ceil(x): smallest int >= x=w231:dbl)
      n169 = Round Toward +Infinity(x=w210) -> (ceil(x): smallest int >= x=w232:dbl)
      n170 = global write "Robot Global Data.vi" "US Raw Left"(w231) -> ()
      n171 = global write "Robot Global Data.vi" "US Raw Right"(w232) -> ()
      n172 = Subtract(x=w210, y=28.0) -> (x-y=w239:dbl)
      n173 = Subtract(x=w211, y=28.0) -> (x-y=w240:dbl)
      n174 = Subtract(x=w211, y=w210) -> (x-y=w216:dbl)
      n175 = Round To Nearest(number=w239) -> (nearest integer value=w238:dbl)
      n176 = Round To Nearest(number=w240) -> (nearest integer value=w237:dbl)
      n177 = global write "Robot Global Data.vi" "US Raw Difference"(w216) -> ()
      n178 = global write "Robot Global Data.vi" "US Gear Right (+)"(w238) -> ()
      n179 = global write "Robot Global Data.vi" "US Gear Left (-)"(w237) -> ()
      n180 = Equal?(x=w238, y=w237) -> (x = y?=w236:bool)
      n181 = Select(t=1.0, s=w236, f=0.0) -> (s? t:f=w235:dbl)
      n182 = global write "Robot Global Data.vi" "US Equality"(w235) -> ()
    }
    frame Enabled {
      n183 = call <vilib>:"WPI_AnalogChannelRefNum Registry Get.vi"("refnum name"="AI 2") -> ("AIDeviceRef"=w250:T17)  [unwired: 9 in, 1 out]
      n184 = call <vilib>:"WPI_AnalogChannelRefNum Registry Get.vi"("refnum name"="AI 1") -> ("AIDeviceRef"=w249:T17)  [unwired: 9 in, 1 out]
      n185 = call <vilib>:"WPI_AnalogChannelGetVoltage.vi"("AIDeviceRef"=w250) -> ("Voltage"=→"Voltage 2":dbl)  [unwired: 8 in, 2 out]
      n186 = call <vilib>:"WPI_AnalogChannelGetVoltage.vi"("AIDeviceRef"=w249) -> ("Voltage"=→"Voltage":dbl)  [unwired: 8 in, 2 out]
    }
  }
  n187 = disable-structure shown="Disabled" {
    frame Disabled {
      n188 = call <vilib>:"WPI_DigitalInputRefNum Registry Get.vi"("refnum name"="Photoeye Front Up") -> ("DigitalInputDevRef"=w266:T19)  [unwired: 9 in, 1 out]
      n189 = call <vilib>:"WPI_DigitalInputRefNum Registry Get.vi"("refnum name"="Photoeye Front Down") -> ("DigitalInputDevRef"=w264:T19)  [unwired: 9 in, 1 out]
      n190 = call <vilib>:"WPI_DigitalInputRefNum Registry Get.vi"("refnum name"="Photoeye Back Up") -> ("DigitalInputDevRef"=w260:T19)  [unwired: 9 in, 1 out]
      n191 = call <vilib>:"WPI_DigitalInputRefNum Registry Get.vi"("refnum name"="Photoeye Back Down") -> ("DigitalInputDevRef"=w261:T19)  [unwired: 9 in, 1 out]
      n192 = call <vilib>:"WPI_DigitalInputRefNum Registry Get.vi"("refnum name"="Gear is Present") -> ("DigitalInputDevRef"=w255:T19)  [unwired: 9 in, 1 out]
      n193 = call <vilib>:"WPI_DigitalInputGetValue.vi"("DigitalInputDevRef"=w255) -> ("Value"=w253:bool)  [unwired: 8 in, 2 out]
      n194 = call <vilib>:"WPI_DigitalInputGetValue.vi"("DigitalInputDevRef"=w266) -> ("Value"=w259:bool)  [unwired: 8 in, 2 out]
      n195 = call <vilib>:"WPI_DigitalInputGetValue.vi"("DigitalInputDevRef"=w264) -> ("Value"=w258:bool)  [unwired: 8 in, 2 out]
      n196 = call <vilib>:"WPI_DigitalInputGetValue.vi"("DigitalInputDevRef"=w260) -> ("Value"=w257:bool)  [unwired: 8 in, 2 out]
      n197 = call <vilib>:"WPI_DigitalInputGetValue.vi"("DigitalInputDevRef"=w261) -> ("Value"=w256:bool)  [unwired: 8 in, 2 out]
      n198 = global write "Robot Global Data.vi" "Photoeye - Back Down"(w256) -> ()
      n199 = global write "Robot Global Data.vi" "Photoeye - Front Up"(w259) -> ()
      n200 = global write "Robot Global Data.vi" "Photoeye - Front Down"(w258) -> ()
      n201 = global write "Robot Global Data.vi" "Photoeye - Back Up"(w257) -> ()
      n202 = global write "Robot Global Data.vi" "Gear is Present (Photoeye)"(w253) -> ()
    }
    frame Enabled {
    }
  }
  n203 = Select(t=120, s=w1, f=15) -> (s? t:f=w4:i32)
  n204 = Select(t=75, s=w1, f=185) -> (s? t:f=w37:i32)
  n205 = call <vilib>:"WPI_SwitchRefNum Registry Get.vi"("refnum name"="Spring Blocked") -> ("SwitchDevRef"=w52:T21)  [unwired: 9 in, 1 out]
  n206 = call <vilib>:"WPI_SwitchRefNum Registry Get.vi"("refnum name"="Top Detect") -> ("SwitchDevRef"=w54:T21)  [unwired: 9 in, 1 out]
  n207 = call <vilib>:"WPI_SwitchRefNum Registry Get.vi"("refnum name"="Spring Penetrate") -> ("SwitchDevRef"=w51:T21)  [unwired: 9 in, 1 out]
  n208 = call <vilib>:"WPI_SwitchGetLimitValue.vi"("SwitchDevRef"=w52) -> ("Switch Pressed"=w49:bool)  [unwired: 8 in, 2 out]
  n209 = call <vilib>:"WPI_SwitchGetLimitValue.vi"("SwitchDevRef"=w54) -> ("Switch Pressed"=w47:bool)  [unwired: 8 in, 2 out]
  n210 = call <vilib>:"WPI_SwitchGetLimitValue.vi"("SwitchDevRef"=w51) -> ("Switch Pressed"=w46:bool)  [unwired: 8 in, 2 out]
  n211 = global write "Robot Global Data.vi" "Limit Switch - Peg Hit Web of Gear (Indicator)"(w49) -> ()
  n212 = global write "Robot Global Data.vi" "Limit Switch - Gear is Present (Indicator)"(w47) -> ()
  n213 = call <vilib>:"WPI_ServoRefNum Registry Get.vi"("refnum name"="Backboard(Left) Servo") -> ("ServoDeviceRef"=w41:T15)  [unwired: 9 in, 1 out]
  n214 = call <vilib>:"WPI_ServoRefNum Registry Get.vi"("refnum name"="Backboard(Right) Servo") -> ("ServoDeviceRef"=w40:T15)  [unwired: 9 in, 1 out]
  n215 = global write "Robot Global Data.vi" "Limit Switch - Peg through Gear (Indicator)"(w46) -> ()
  n216 = call <vilib>:"WPI_ServoSetAngle.vi"("Angle"=w4, "ServoDeviceRef"=w41) -> ()  [unwired: 8 in, 2 out]
  n217 = call <vilib>:"WPI_ServoSetAngle.vi"("Angle"=w37, "ServoDeviceRef"=w40) -> ()  [unwired: 8 in, 2 out]
  n218 = disable-structure shown="Disabled" {
    frame Disabled {
      n219 = global read "Robot Global Data.vi" "Gear Flip Servo"() -> (w274:bool)
      n220 = feedback #4() -> (w276:bool)  [unwired: 1 in]
      n221 = feedback-in #4(w274) -> ()
      n222 = Greater?(x=w274, y=w276) -> (0:w275:bool)
      n223 = case shown="True" w275 {
        tunnel: [w277 w278] -> w273
        frame False {
          n224 = local read "Toggle 7"() -> (w277:bool)
        }
        frame True {
          n225 = local read "Toggle 7"() -> (w279:bool)
          n226 = Not(x=w279) -> (.not. x?=w278:bool)
          n227 = local write "Toggle 7"(w278) -> ()
        }
      }
      n228 = Select(t=180.0, s=w273, f=0.0) -> (s? t:f=w268:dbl)
      n229 = call <vilib>:"WPI_ServoRefNum Registry Get.vi"("refnum name"="Gear Flip Servo") -> ("ServoDeviceRef"=w269:T15)  [unwired: 9 in, 1 out]
      n230 = call <vilib>:"WPI_ServoSetAngle.vi"("Angle"=w268, "ServoDeviceRef"=w269) -> ()  [unwired: 8 in, 2 out]
    }
    frame Enabled {
    }
  }
